vi "FPGA cRIOMain_v4.vi"() -> ()   [LabVIEW 2019]
doc: "Main FPGA VI\nUse the bitfile generated by this VI in the real-time code.\n\nFlip the channels for input and output"
uses:
  TypeDefs/AO mode TabCtrl.ctl
  TypeDefs/SamplingModeEnum.ctl
  TypeDefs/AI_channelEnum.ctl
  <vilib>/rvi/Emulation/niFpgaGetClockAttributes.vi
  <vilib>/rvi/Emulation/niFpgaSctlEmulationGetInTimedLoop.vi
  <vilib>/rvi/Emulation/niFpgaEmulationReportErrorSimple.vi
  <vilib>/rvi/eio/common/nirviEmuTemplateMethod_errors.vi
  <vilib>/rvi/Emulation/niFpgaProcessEmulError.vi
  <vilib>/rvi/Emulation/niFpgaCriticalErrorInLSC.vi
  <vilib>/rvi/Emulation/niFpgaEmulationIsFPGAContextNoSignature.vi
  <vilib>/rvi/errors/niFpgaSetErrorForExecOnDevCompSimple.vi
  <vilib>/rvi/eio/common/nirviEmuReportErrorAndStop.vi
  <vilib>/rvi/DataTransferAndStorage/Container/Common/niFpgaContainerGetUniqueNameForEmu.vi
  <vilib>/rvi/FIFO/Fifo_Resource/nirvififoEmulationSetSize.vi
  <vilib>/rvi/FIFO/Fifo_Resource/nirviFifoEmulationQueueMgr.vi
  <instcachedir>/0/nirviFifoEmulationQueueMgr_E5CAEC123FF24DC58D834DCA3CDAA9B5.lvgen/nirviFifoEmulationQueueMgr_E5CAEC123FF24DC58D834DCA3CDAA9B5_006.vi
  <vilib>/Utility/error.llb/Clear Errors.vi
  <vilib>/rvi/FIFO/Fifo_Resource/nirvififoEmulationCreateLock.vi
  <vilib>/rvi/FIFO/Fifo_Resource/nirvififoEmulationObtainLock.vi
  <vilib>/rvi/FIFO/Fifo_Resource/nirvififoEmulationReleaseLock.vi
  <vilib>/rvi/occurrence/nirviWaitOnOccurrenceBase.vi
  <vilib>/rvi/errors/nirviReportUnexpectedCaseInternalError.vi
  <vilib>/rvi/errors/nirviReportUnexpectedCaseInternalError (U32).vi
  <vilib>/rvi/FIFO/Fifo_Resource/nirvififoEmulationDetermineInputValidOut.vi
  <vilib>/eio/EIONode/EIONode.xnode
  <vilib>/rvi/DataTransferAndStorage/Container/XNode/niFpgaContainer.xnode
  <vilib>/rvi/FIFO/Fifo_Resource/nirvififoEmulationRead.vi
  <vilib>/rvi/Analysis/measure/butterworth/XNode/niFpgaButterworthFilter.xnode
  <vilib>/rvi/FXPMathLib/FxpMul/XNode/nifxpmath_Multiplier.xnode
  <vilib>/rvi/FIFO/Fifo_Resource/nirvififoEmulationWrite.vi
  FPGA functions/FPGA functions.lvlib
  <vilib>/rvi/FXPMathLib/sim/FxpSim.dll
panel:
  out "AI Processing\nLoop Rate to high?":bool
  in  "AI Process Time [ticks]":u32=120
  in  "Select Channel":T1
  out "Unable to\nsample at desired\nSample Rate?":bool
  out "Processing Loop time [ticks]":u32
  in  "Scaled Butterworth Coeffs":i32[](array[numeric])=[-1036986264, 2110353124, 93741, -1058362983, 2131726043, 94691]
  in  "Sampling Mode":T2
  in  "AO mode":T3
  in  "AO Out [V]":fxp<+/-,18,5> format="%#.6g"
  in  "AO enable?":bool
  out "AI In [V]":fxp<+/-,25,5> format="%#.6g"
  out "FPGA AO DMA\nOverflow?":bool
  out "Int. Output":fxp<+/-,20,5> format="%.17g"
  out "Raw Int. Input":fxp<+/-,24,5> format="%.21g"
  in  "Sample Time [ticks]":u32=120
  out "AO Loop time [ticks]":u32
  out "AI Loop time [ticks]":u32
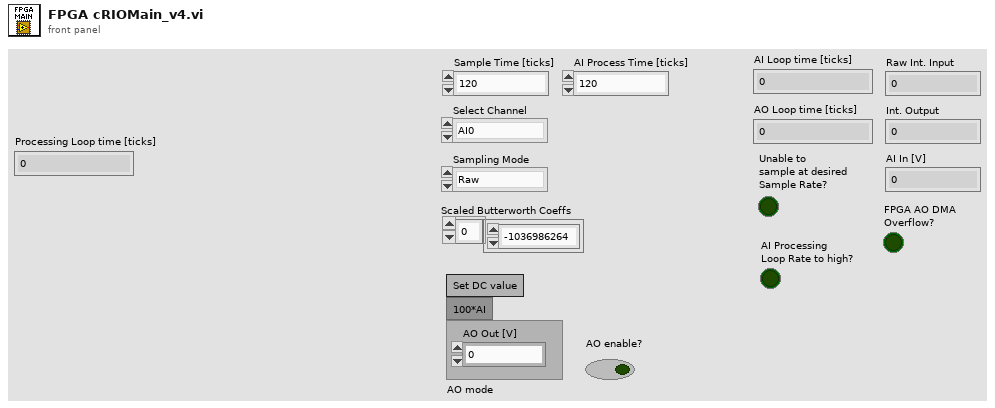
[diagram p1: front panel]
types:
  T1 = typedef "AI_channelEnum.ctl" = enum16{"AI0", "AI1", "AI2", "AI3"}
  T2 = typedef "SamplingModeEnum.ctl" = enum16{"Raw", "LPF", "4 pt. Avg. + LPF"}
  T3 = typedef "AO mode TabCtrl.ctl" = enum32{"Set DC value", "100*AI"}
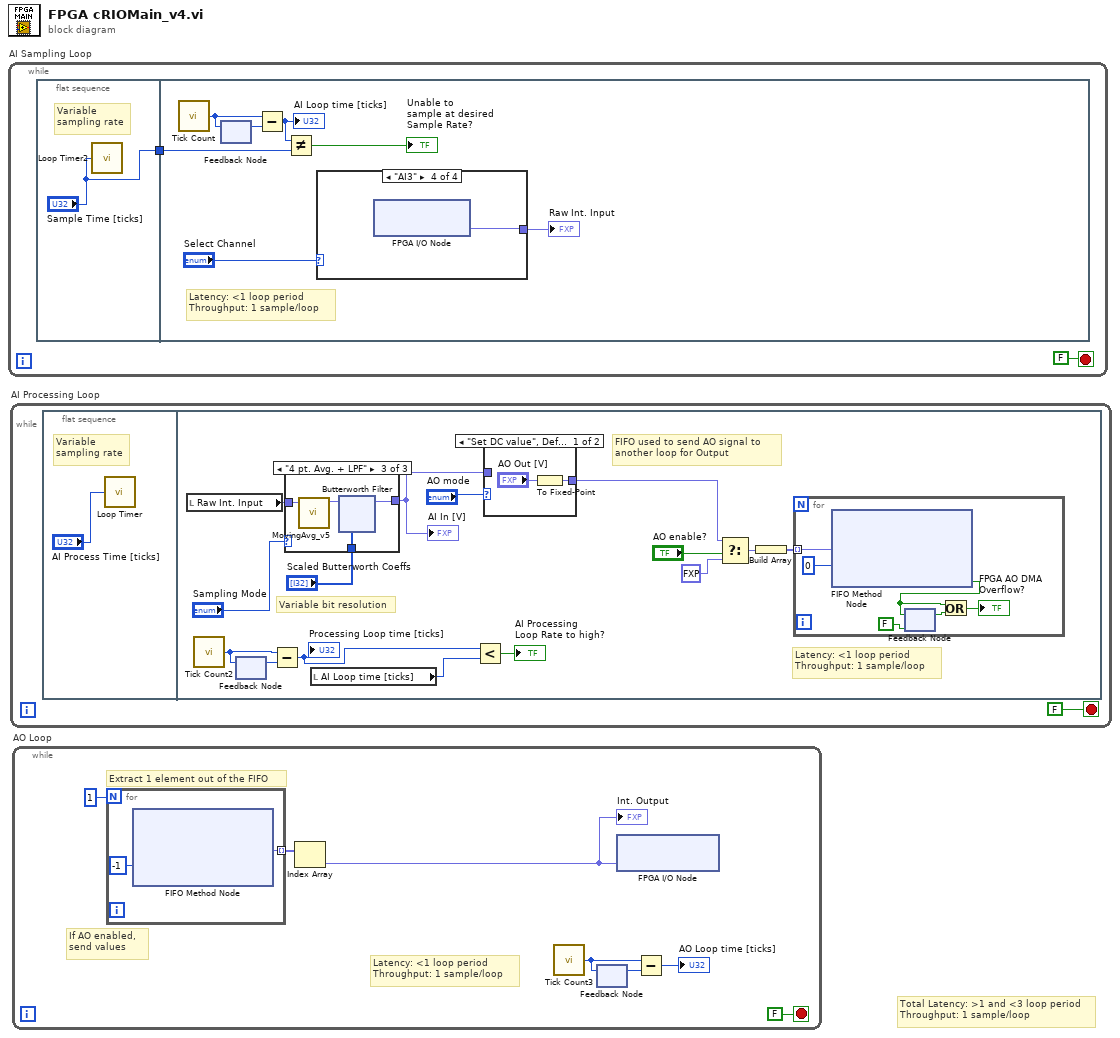
[diagram p0: block diagram]
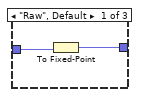
[diagram p2: hidden frame]
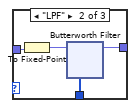
[diagram p3: hidden frame]
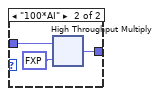
[diagram p4: hidden frame]
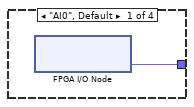
[diagram p5: hidden frame]
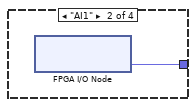
[diagram p6: hidden frame]
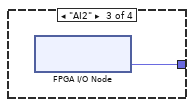
[diagram p7: hidden frame]
diagram:
  # "Total Latency: >1 and <3 loop period\nThroughput: 1 sample/loop"
  n1 = while "AI Sampling Loop" {
    stop <- FALSE stop-if-true
    n2 = flat-sequence {
      tunnel: ["Sample Time [ticks]"] -> w1
      tunnel: w1 -> [w7]
      frame #0 {
        # "Variable\nsampling rate"
        n3 = call "Loop Timer2"("Count(Ticks)"="Sample Time [ticks]") -> ()  [unwired: 1 out]
      }
      frame #1 {
        # "Latency: <1 loop period\nThroughput: 1 sample/loop"
        n4 = call "Tick Count"() -> ("Tick Count(Ticks)"=w10:u32)
        n5 = feedback #1() -> (w9:u32)  [unwired: 1 in]
        n6 = feedback-in #1(w10) -> ()
        n7 = Subtract(x=w10, y=w9) -> (x-y=w8:u32)
        "AI Loop time [ticks]" <- w8
        n8 = Not Equal?(x=w8, y=w7) -> (x != y?=→"Unable to\nsample at desired\nSample Rate?":bool)
        n9 = case shown="\"AI3\"" "Select Channel" {
          tunnel: [w11 w12 w13 w14] -> w4
          frame "AI0", Default {
            n10 = xnode "FPGA I/O Node"() -> ("Mod4/AI0"=w11:fxp<+/-,24,5>)  [unwired: 1 in, 1 out]
          }
          frame "AI1" {
            n11 = xnode "FPGA I/O Node"() -> ("Mod4/AI1"=w12:fxp<+/-,24,5>)  [unwired: 1 in, 1 out]
          }
          frame "AI2" {
            n12 = xnode "FPGA I/O Node"() -> ("Mod4/AI2"=w13:fxp<+/-,24,5>)  [unwired: 1 in, 1 out]
          }
          frame "AI3" {
            n13 = xnode "FPGA I/O Node"() -> ("Mod4/AI3"=w14:fxp<+/-,24,5>)  [unwired: 1 in, 1 out]
          }
        }
        "Raw Int. Input" <- w4
      }
    }
  }
  n14 = while "AI Processing Loop" {
    stop <- FALSE stop-if-true
    n15 = flat-sequence {
      frame #0 {
        # "Variable\nsampling rate"
        n16 = call "Loop Timer"("Count(Ticks)"="AI Process Time [ticks]") -> ()  [unwired: 1 out]
      }
      frame #1 {
        # "Variable bit resolution"
        # "Latency: <1 loop period\nThroughput: 1 sample/loop"
        # "FIFO used to send AO signal to \nanother loop for Output"
        n17 = local read "Raw Int. Input"() -> (w18:fxp<+/-,24,5>)
        n18 = call "Tick Count2"() -> ("Tick Count(Ticks)"=w30:u32)
        n19 = feedback #2() -> (w31:u32)  [unwired: 1 in]
        n20 = feedback-in #2(w30) -> ()
        n21 = Subtract(x=w30, y=w31) -> (x-y=w20:u32)
        "Processing Loop time [ticks]" <- w20
        n22 = case shown="\"4 pt. Avg. + LPF\"" "Sampling Mode" {
          tunnel: "Scaled Butterworth Coeffs" -> [_ w37 w49]
          tunnel: [w33 w36 w48] -> w28
          tunnel: w18 -> [w32 w34 w46]
          frame "Raw", Default {
            n23 = To Fixed-Point(number=w32) -> (fixed-point=w33:fxp<+/-,25,5>)  [unwired: 1 in]
          }
          frame "LPF" {
            n24 = To Fixed-Point(number=w34) -> (fixed-point=w35:fxp<+/-,25,5>)  [unwired: 1 in]
            n25 = xnode "Butterworth Filter"("input data"=w35, "scaled coefficients"=w37) -> ("output data"=w36:fxp<+/-,25,5>)  [unwired: 1 in]
          }
          frame "4 pt. Avg. + LPF" {
            n26 = call "MovingAvg_v5.vi"("Raw input"=w46) -> ("Avg. output"=w47:fxp<+/-,25,5>)  [unwired: 10 in]
            n27 = xnode "Butterworth Filter"("input data"=w47, "scaled coefficients"=w49) -> ("output data"=w48:fxp<+/-,25,5>)  [unwired: 1 in]
          }
        }
        "AI In [V]" <- w28
        n28 = local read "AI Loop time [ticks]"() -> (w19:u32)
        n29 = Less?(x=w20, y=w19) -> (x < y?=→"AI Processing\nLoop Rate to high?":bool)
        n30 = case shown="\"Set DC value\", Default" "AO mode" {
          tunnel: [w59 w60] -> w24
          tunnel: w28 -> [_ w62]
          frame "Set DC value", Default {
            n31 = To Fixed-Point(number="AO Out [V]") -> (fixed-point=w59:fxp<+/-,20,5>)  [unwired: 1 in]
          }
          frame "100*AI" {
            n32 = xnode ("High Throughput Multiply")("x"=w62, "y"=fxp<+,5,7> 100.0) -> ("x*y"=w60:fxp<+/-,20,5>)
          }
        }
        n33 = Select(t=w24, s="AO enable?", f=fxp<+/-,20,5> 0.0) -> (s? t:f=w29:fxp<+/-,20,5>)
        n34 = Build Array(w29) -> (w23:fxp<+/-,20,5>[])
        n35 = for {
          tunnel: w23 -> [w63] mode=indexing
          n36 = xnode ("FIFO Method Node")("Element"=w63, "Timeout"=0) -> ("Timed Out?"=w64:bool)  [unwired: 1 in, 1 out]
          n37 = feedback-in #3(w64) -> ()
          n38 = feedback #3(FALSE ("Timed Out?")) -> (w67:bool)
          n39 = Or(x=w64, y=w67) -> (x .or. y?=→"FPGA AO DMA\nOverflow?":bool)
        }
      }
    }
  }
  n40 = while "AO Loop" {
    stop <- FALSE stop-if-true
    # "Latency: <1 loop period\nThroughput: 1 sample/loop"
    # "If AO enabled, \nsend values"
    # "Extract 1 element out of the FIFO"
    n41 = for {
      N: 1 -> [_]
      tunnel: [w77] -> w71 mode=indexing
      n42 = xnode ("FIFO Method Node")("Timeout"=-1) -> ("Element"=w77:fxp<+/-,20,5>)  [unwired: 1 in, 2 out]
    }
    n43 = Index Array(array=w71) -> (element=w69:fxp<+/-,20,5>)  [unwired: 1 in]
    "Int. Output" <- w69
    n44 = call "Tick Count3"() -> ("Tick Count(Ticks)"=w74:u32)
    n45 = feedback #4() -> (w73:u32)  [unwired: 1 in]
    n46 = feedback-in #4(w74) -> ()
    n47 = xnode "FPGA I/O Node"("Mod3/AO1"=w69) -> ()  [unwired: 1 in, 1 out]
    n48 = Subtract(x=w74, y=w73) -> (x-y=→"AO Loop time [ticks]":u32)
  }
